vi "4.3.1.vi"() -> ()   [LabVIEW 2018]
panel:
  out "숫자형":dbl
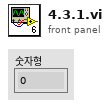
[diagram p1: front panel]
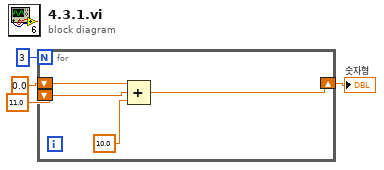
[diagram p0: block diagram]
diagram:
  n1 = for {
    N: 3 -> [_]
    shift-right: [w7] -> w3
    shift-left: 0.0 -> [w8]
    shift-left: 11.0 -> [w6]
    n2 = Compound Arithmetic op=ADD(w8, w6, 10.0 ("값")) -> (w7:dbl)
  }
  "숫자형" <- w3
